vi "Initialize.vi"(0 "Interface in":T1, 5 "numOfInterleaves":u8, 7 "rampRate":sgl format="%#_13g", 9 "gains":T3 {"proportional gain" step=0.125}, 11 "error in":errorcluster, 12 "modulationConfig":T2 {"modulationRate" format="%#_6p"; "Deadband" format="%#_6p"; "SwitchingSpeed" format="%#_6p"}) -> (4 "Interface out":T1, 15 "error out":errorcluster)   [LabVIEW 2017, in "BuckBoostInterface.lvlib"]
uses:
  BuckBoostInterface.lvlib
  Interface.ctl
  <instrlib>/_niInstr/Instruction Framework/v1/Host/Instruction Target/niInstr Instruction Target v1 Host.lvclass
  <instrlib>/_niInstr/Instruction Framework/v1/Host/Instruction Framework Context/niInstr Instruction Framework Context v1 Host.lvclass
  <vilib>/rvi/Analysis/control/PID/Typedef/niFpgaPID_PIGains.ctl
  modulationConfig.ctl
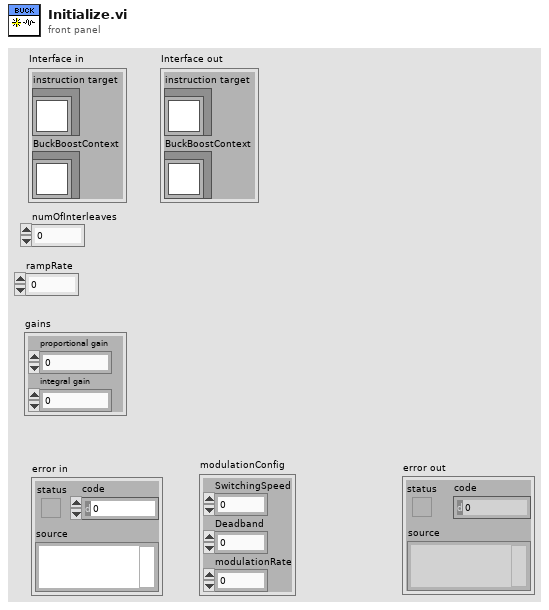
[diagram p1: front panel]
types:
  T1 = typedef "BuckBoostInterface.lvlib/Interface.ctl" = cluster{"instruction target":refnum<class "niInstr Instruction Target v1 Host.lvclass">, "BuckBoostContext":refnum<class "niInstr Instruction Framework Context v1 Host.lvclass">}
  T2 = typedef "BuckBoostInterface.lvlib/modulationConfig.ctl" = cluster{"SwitchingSpeed":dbl, "Deadband":dbl, "modulationRate":dbl}
  T3 = typedef "niFpgaPID_PIGains.ctl" = cluster{"proportional gain":sgl, "integral gain":sgl}
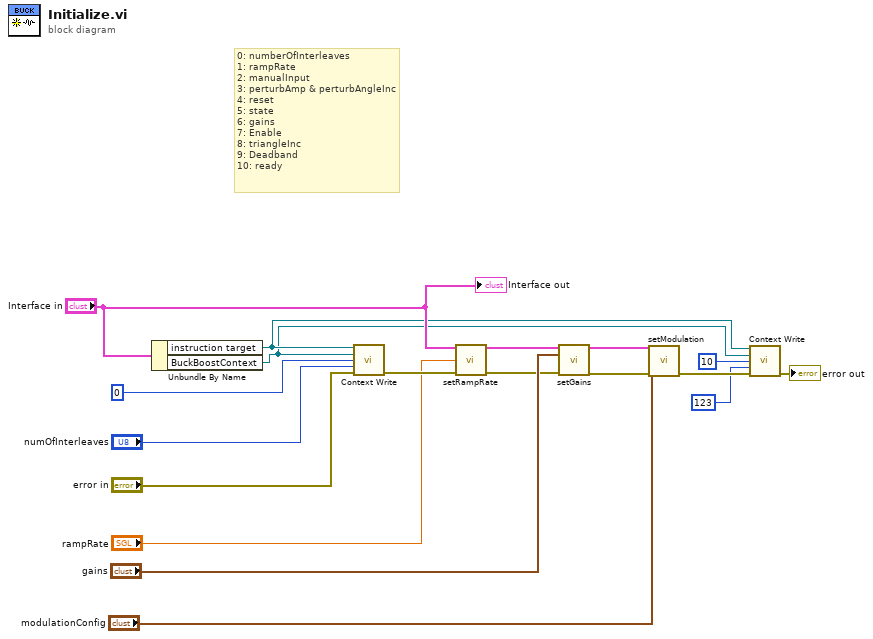
[diagram p0: block diagram]
diagram:
  # "0: numberOfInterleaves\n1: rampRate\n2: manualInput\n3: perturbAmp & perturbAngleInc\n4: reset\n5: state\n6: gains\n7: Enable\n8: triangleInc\n9: Deadband\n10: ready"
  n1 = Unbundle By Name("Interface in") -> ("instruction target"=w6:refnum<class "niInstr Instruction Target v1 Host.lvclass">, "BuckBoostContext"=w5:refnum<class "niInstr Instruction Framework Context v1 Host.lvclass">)
  n2 = call <instrlib>:"Context Write.vi"("instruction target in"=w6, "context in"=w5, "address"=u64 0, "data"="numOfInterleaves", "error in"="error in") -> ("error out"=w15:errorcluster)  [unwired: 8 in, 2 out]
  n3 = call "setRampRate.vi"("Interface in"="Interface in", "rampRate"="rampRate", "error in (no error)"=w15) -> ("Interface out"=w11:T1, "error out"=w10:errorcluster)  [unwired: 11 in]
  n4 = call "setGains.vi"("Interface in"=w11, "gains"="gains", "error in (no error)"=w10) -> ("Interface out"=w9:T1, "error out"=w8:errorcluster)  [unwired: 11 in]
  n5 = call "setModulation.vi"("Interface in"=w9, "modulationConfig"="modulationConfig", "error in (no error)"=w8) -> ("error out"=w4:errorcluster)  [unwired: 11 in, 1 out]
  n6 = call <instrlib>:"Context Write.vi"("instruction target in"=w6, "context in"=w5, "address"=u64 10, "data"=u64 123, "error in"=w4) -> ("error out"=→"error out":errorcluster)  [unwired: 8 in, 2 out]
  "Interface out" <- "Interface in"
